vi "Disconnect.vi"(8 "error in":errorcluster, 11 "336XX in":refnum<class "336XX.lvclass">) -> (0 "error out":errorcluster, 3 "336XX out":refnum<class "336XX.lvclass">)   [LabVIEW 2019, in "336XX.lvlib" / "336XX.lvclass"]
uses:
  Library/336XX.lvclass
  Library/336XX.lvclass/336XX.ctl
  builds/Instruments/FunctionGenerator.lvlibp/Library/FunctionGenerator.lvclass
  <instrlib>/Agilent 3352X Series/Agilent 3352X Series.lvlib
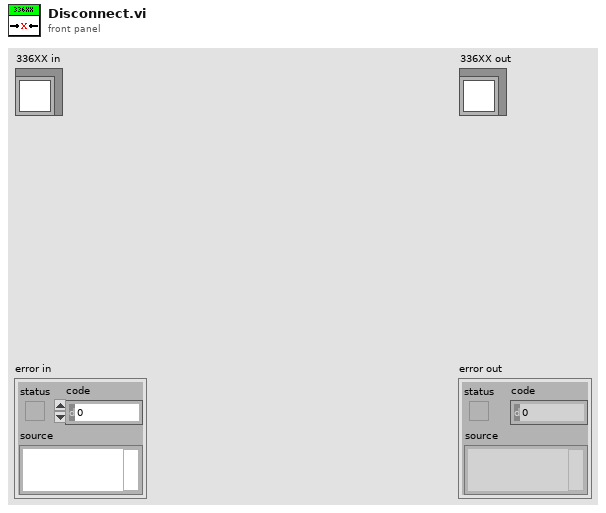
[diagram p1: front panel]
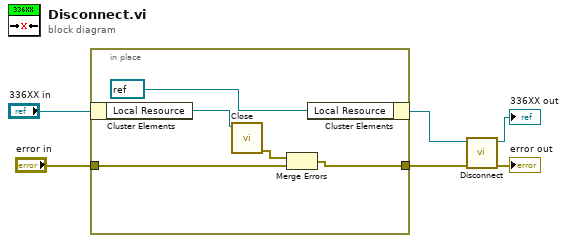
[diagram p0: block diagram]
diagram:
  n1 = in-place {
    in-place-border: "error in" -> [w9]
    in-place-border: [w8] -> w2
    n2 = in-place-cluster #1("336XX in") -> ("Local Resource"=w11:refnum<visa-resource-name>)
    n3 = call <instrlib>:"Close.vi"("VISA resource name"=w11) -> ("error out"=w10:errorcluster)  [unwired: 10 in]
    n4 = Merge Errors(w10, w9) -> (w8:errorcluster)
    n5 = in-place-cluster #1("Local Resource"=refnum<visa-resource-name> refnum) -> (w1:refnum<class "336XX.lvclass">)
  }
  n6 = call-parent "Disconnect.vi"("error in"=w2, "FunctionGenerator in"=w1) -> ("error out"=→"error out":errorcluster, "FunctionGenerator out"=→"336XX out":refnum<class "336XX.lvclass">)  [unwired: 8 in]
